vi "Divide.vi"(0 "num_1":dbl, 5 "num_2":dbl) -> (4 "result":dbl)   [LabVIEW 2023]
doc: "Divide two numbers (Double)"
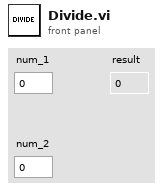
[diagram p1: front panel]
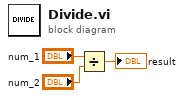
[diagram p0: block diagram]
diagram:
  n1 = Divide(x="num_1", y="num_2") -> (x/y=→"result":dbl)
